vi "fitFocus.vi"(8 "error in (no error)":errorcluster, 9 "num_measurements":i32, 10 "heights":dbl[](array[numeric]), 11 "focus_values":dbl[](array[numeric])) -> (0 "error out":errorcluster, 2 "focus height":dbl)   [LabVIEW 2011, in "gVision.lvlib"]
uses:
  gVision.lvlib
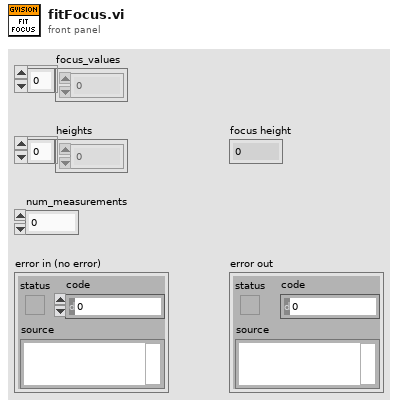
[diagram p1: front panel]
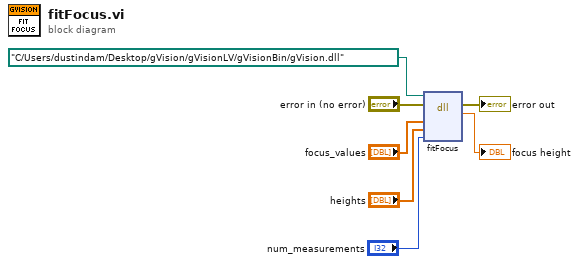
[diagram p0: block diagram]
diagram:
  n1 = dll-call lib="C:/Users/Husker/Desktop/gantry/gVision/Release/gVision.dll" fn="fitFocus"(path in=path "C:/Users/dustindam/Desktop/gVision/gVisionLV/gVisionBin/gVision.dll", error in="error in (no error)", "focus_values"="focus_values", "heights"="heights", "num_measurements"="num_measurements") -> (error out=→"error out":errorcluster, "return type"=→"focus height":dbl)  [unwired: 4 in, 1 out]
